vi "Init.vi"(8 "error in (no error)":errorcluster, 11 "DLL Path (Auto)":path) -> (0 "error out":errorcluster, 2 "Running?":bool, 3 "VoiceMeeterRemote out":refnum<class "VoiceMeeterRemote.lvclass">)   [LabVIEW 2020, in "VoiceMeeterRemote.lvlib" / "VoiceMeeterRemote.lvclass"]
doc: "Initializes the VMR API instance and returns whether Voicemeeter is already running or not.\n\n<b>DLL Path</b> can be left unwired if Voicemeeter was installed to the default location. If Voicemeeter was installed to a different path then the location to the VoiceMeeterRemote.dll or VoiceMeeterRemote64.dll must be provided."
uses:
  VoiceMeeterRemote.lvclass
  VoiceMeeterRemote.lvlib
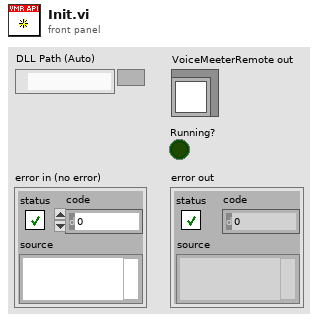
[diagram p1: front panel]
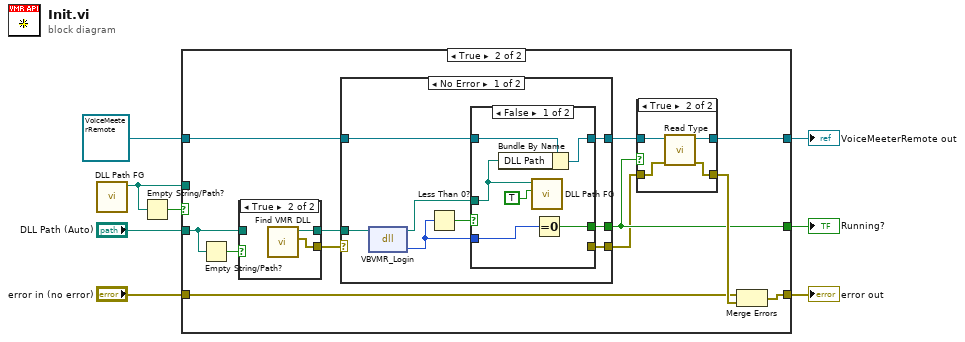
[diagram p0: block diagram]
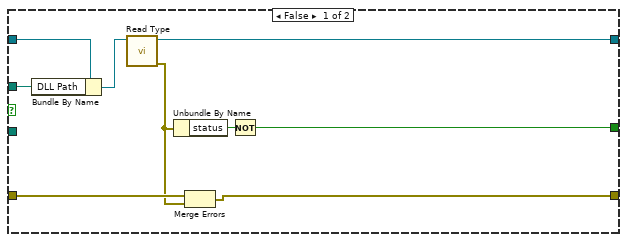
[diagram p2: hidden frame]
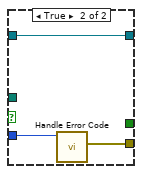
[diagram p4: hidden frame]
diagram:
  n1 = call "DLL Path FG.vi"() -> ("DLL Path"=w2:path)  [unwired: 11 in]
  n2 = Empty String/Path?(string/path=w2) -> (empty?=w3:bool)
  n3 = case shown="True" w3 {
    tunnel: "error in (no error)" -> [w11 w28]
    tunnel: "DLL Path (Auto)" -> [_ w26]
    tunnel: [w9 w23] -> w6
    tunnel: [w14 w19] -> w5
    tunnel: [w12 w20] -> w4
    tunnel: w2 -> [w16 _]
    tunnel: refnum<class "VoiceMeeterRemote.lvclass"> refnum ("VoiceMeeterRemote in") -> [w17 w22]
    frame False {
      n4 = Bundle By Name(cluster=w17, "DLL Path"=w16) -> (w15:refnum<class "VoiceMeeterRemote.lvclass">)
      n5 = call "Read Type.vi"("VoiceMeeterRemote in"=w15) -> ("error out"=w10:errorcluster, "VoiceMeeterRemote out"=w14:refnum<class "VoiceMeeterRemote.lvclass">)  [unwired: 9 in]
      n6 = Unbundle By Name(w10) -> ("status"=w13:bool)
      n7 = Merge Errors(w11, w10) -> (w9:errorcluster)
      n8 = Not(x=w13) -> (.not. x?=w12:bool)
    }
    frame True {
      n9 = Empty String/Path?(string/path=w26) -> (empty?=w27:bool)
      n10 = case shown="True" w27 {
        tunnel: w26 -> [w55 _]
        tunnel: [w55 w57] -> w25
        tunnel: [_ w56] -> w24
        frame False {
        }
        frame True {
          n11 = call "Find VMR DLL.vi"() -> ("error out"=w56:errorcluster, "DLL Path"=w57:path)  [unwired: 10 in]
        }
      }
      n12 = case shown="No Error" w24 {
        selector: w24 -> [_ w54]
        tunnel: w25 -> [w43 _]
        tunnel: [w37 w54] -> w18
        tunnel: w22 -> [w42 w53]
        tunnel: [w38 w53] -> w21
        tunnel: [w36 _] -> w20
        frame No Error {
          n13 = dll-call lib="C:/Program Files/National Instruments/LabVIEW 2022/user.lib/VoicemeeterRemote64/VoicemeeterRemote64.*" fn="VBVMR_Login"(path in=w43) -> (path out=w41:path, "return type"=w39:i32)  [unwired: 2 in, 1 out]
          n14 = Less Than 0?(x=w39) -> (x < 0?=w40:bool)
          n15 = case shown="False" w40 {
            tunnel: w42 -> [w49 w52]
            tunnel: w41 -> [w45 _]
            tunnel: w39 -> [w47 w51]
            tunnel: [w48 w52] -> w38
            tunnel: [_ w50] -> w37
            tunnel: [w46 _] -> w36
            frame False {
              n16 = Bundle By Name(cluster=w49, "DLL Path"=w45) -> (w48:refnum<class "VoiceMeeterRemote.lvclass">)
              n17 = call "DLL Path FG.vi"("Set? (F)"=TRUE, "DLL Path In"=w45) -> ()  [unwired: 9 in, 1 out]
              n18 = Equal To 0?(x=w47) -> (x = 0?=w46:bool)
            }
            frame True {
              n19 = call "Handle Error Code.vi"("Code"=w51) -> ("error out"=w50:errorcluster)  [unwired: 10 in]
            }
          }
        }
        frame Error {
        }
      }
      n20 = case shown="True" w20 {
        tunnel: w21 -> [w30 w35]
        tunnel: [w30 w34] -> w19
        tunnel: w18 -> [w31 w33]
        tunnel: [w31 w32] -> w29
        frame False {
        }
        frame True {
          n21 = call "Read Type.vi"("error in (no error)"=w33, "VoiceMeeterRemote in"=w35) -> ("error out"=w32:errorcluster, "VoiceMeeterRemote out"=w34:refnum<class "VoiceMeeterRemote.lvclass">)  [unwired: 8 in]
        }
      }
      n22 = Merge Errors(w28, w29) -> (w23:errorcluster)
    }
  }
  "error out" <- w6
  "VoiceMeeterRemote out" <- w5
  "Running?" <- w4
